vi "setUp.vi"(8 "error in (no error)":errorcluster, 11 "reference in":refnum<class "DMA Channels Basic Testing.lvclass">) -> (0 "error out":errorcluster, 3 "reference out":refnum<class "DMA Channels Basic Testing.lvclass">)   [LabVIEW 2019, in "DMA Channels Basic Testing.lvclass"]
doc: "setUp runs prior to the test method during test execution. Use this method to initialize any object data required by your tests."
uses:
  DMA Channels Basic Testing.lvclass
  C:/Users/dstavila/Desktop/FPGA Addon Custom Device Main/Source/Tests/FPGA Addon Test Class/FPGA Addon Test Class.lvclass
  FPGA Addon Test Class/FPGA Addon Test Class.lvclass/FPGA Addon Test Class.ctl
  4cbd2b1b-ede0-4ec4-b8d7-c7235fc19dc4.vi
  FPGA Addon Test Class/FPGA Addon Test Class.lvclass
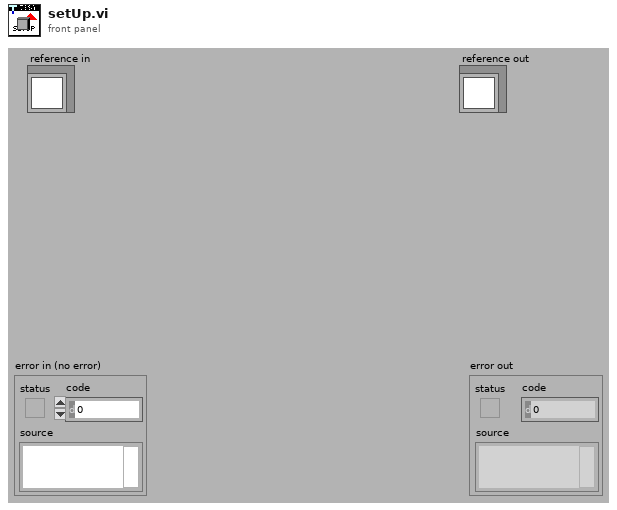
[diagram p1: front panel]
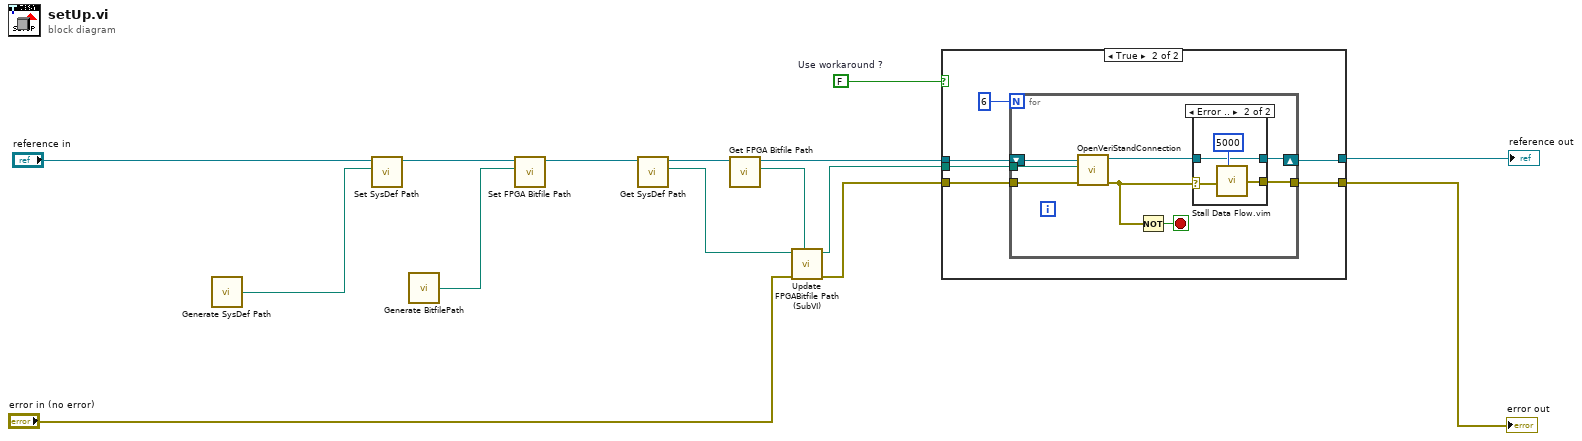
[diagram p0: block diagram]
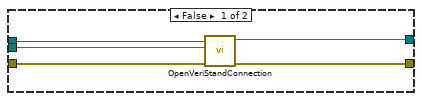
[diagram p2: hidden frame]
diagram:
  w1 = FALSE  # Use workaround ?
  n1 = call "Generate SysDef Path.vi"() -> ("SysDef path"=w9:path)
  n2 = call "Set SysDef Path.vi"("SysDef Path"=w9, "Scalar Channels Testing in"="reference in") -> ("Scalar Channels Testing out"=w15:refnum<class "DMA Channels Basic Testing.lvclass">)  [unwired: 9 in]
  n3 = call "Generate BitfilePath.vi"() -> ("Bitfile path"=w8:path)
  n4 = call "Set FPGA Bitfile Path.vi"("FPGA Bitfile Path"=w8, "Scalar Channels Testing in"=w15) -> ("Scalar Channels Testing out"=w14:refnum<class "DMA Channels Basic Testing.lvclass">)  [unwired: 9 in]
  n5 = call "Get SysDef Path.vi"("Scalar Channels Testing in"=w14) -> ("SysDef Path"=w11:path, "Scalar Channels Testing out"=w13:refnum<class "DMA Channels Basic Testing.lvclass">)  [unwired: 9 in]
  n6 = call "Get FPGA Bitfile Path.vi"("Scalar Channels Testing in"=w13) -> ("FPGA Bitfile Path"=w12:path, "Scalar Channels Testing out"=w6:refnum<class "DMA Channels Basic Testing.lvclass">)  [unwired: 9 in]
  n7 = call "Update FPGABitfile Path (SubVI).vi"("Bitfile Path"=w12, "error in (no error)"="error in (no error)", "System Definition path in"=w11) -> ("error out"=w5:errorcluster, "System Definition path out"=w3:path)  [unwired: 7 in]
  n8 = case shown="True" w1 {
    tunnel: w6 -> [w20 w25]
    tunnel: w5 -> [w19 w23]
    tunnel: [w18 w24] -> w4
    tunnel: w3 -> [w17 w21]
    tunnel: [w16 w22] -> w2
    frame False {
      n9 = call-dynamic "OpenVeriStandConnection.vi"("error in (no error)"=w19, "System Definition File"=w17, "VeriStand Test Case in"=w20) -> ("error out"=w16:errorcluster, "VeriStand Test Case out"=w18:refnum<class "DMA Channels Basic Testing.lvclass">)  [unwired: 6 in, 1 out]
    }
    frame True {
      n10 = for {
        N: 6 -> [_]
        shift-right: [w28] -> w24
        shift-left: w25 -> [w34]
        tunnel: [w33] -> w22
        tunnel: w23 -> [w32]
        tunnel: w21 -> [w31]
        stop <- w27 stop-if-true
        n11 = call-dynamic "OpenVeriStandConnection.vi"("error in (no error)"=w32, "System Definition File"=w31, "VeriStand Test Case in"=w34) -> ("error out"=w30:errorcluster, "VeriStand Test Case out"=w29:refnum<class "DMA Channels Basic Testing.lvclass">)  [unwired: 6 in, 1 out]
        n12 = Not(x=w30) -> (.not. x?=w27:bool)
        n13 = case shown="Error .." w30 {
          selector: w30 -> [w36 w38]
          tunnel: [w36 w40] -> w33
          tunnel: w29 -> [w35 w37]
          tunnel: [w35 w37] -> w28
          frame No Error {
          }
          frame Error {
            n14 = call "Stall Data Flow.vim"("value in"=w38, "milliseconds to wait"=u32 5000) -> ("value out"=w40:errorcluster)  [unwired: 1 out]
          }
        }
      }
    }
  }
  "error out" <- w2
  "reference out" <- w4
